vi "Recording_Main.vi"(8 "error in":errorcluster, 11 "QRD":T1) -> (0 "error out":errorcluster)   [LabVIEW 2025]
uses:
  Builds/Queue Wrappers.lvlibp
  Controls/Local Data_Recording.ctl
  Builds/Queue Wrappers.lvlibp/Q Packet.ctl
  Controls/Queues-Refs-Data.ctl
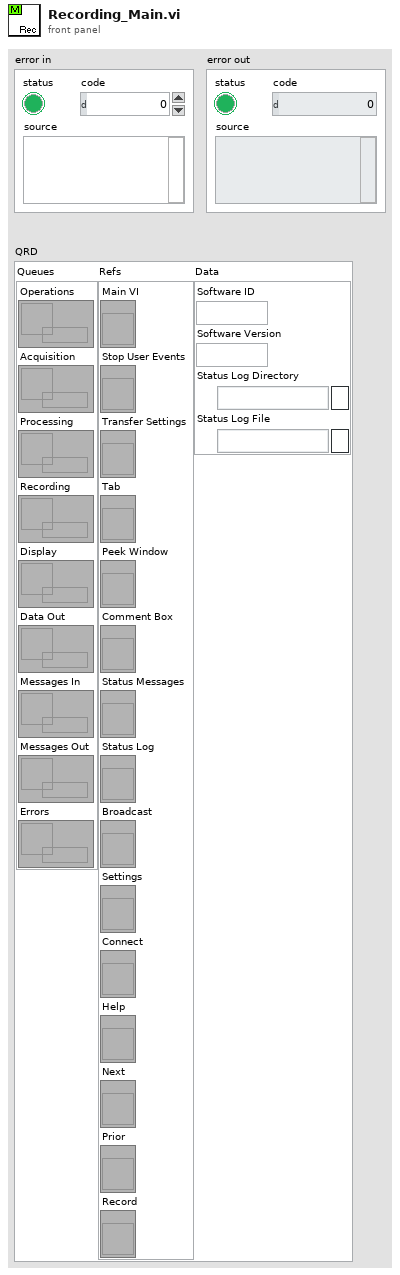
[diagram p1: front panel]
types:
  T1 = typedef "Queues-Refs-Data.ctl" = cluster{"Queues":cluster{"Operations":refnum<queue>, "Acquisition":refnum<queue>, "Processing":refnum<queue>, "Recording":refnum<queue>, "Display":refnum<queue>, "Data Out":refnum<queue>, "Messages In":refnum<queue>, "Messages Out":refnum<queue>, "Errors":refnum<queue>}, "Refs":cluster{"Main VI":refnum<vi>, "Stop User Events":refnum<vi>, "Transfer Settings":refnum<vi>, "Tab":refnum<vi>, "Peek Window":refnum<vi>, "Comment Box":refnum<vi>, "Status Messages":refnum<vi>, "Status Log":refnum<vi>, "Broadcast":refnum<vi>, "Settings":refnum<vi>, "Connect":refnum<vi>, "Help":refnum<vi>, "Next":refnum<vi>, "Prior":refnum<vi>, "Record":refnum<vi>}, "Data":cluster{"Software ID":string, "Software Version":string, "Status Log Directory":path, "Status Log File":path}}
  T2 = typedef "Local Data_Recording.ctl" = cluster{"Loop ID":string, "Output Dir":path, "Output File":path, "Output File Ref":refnum<k34>}
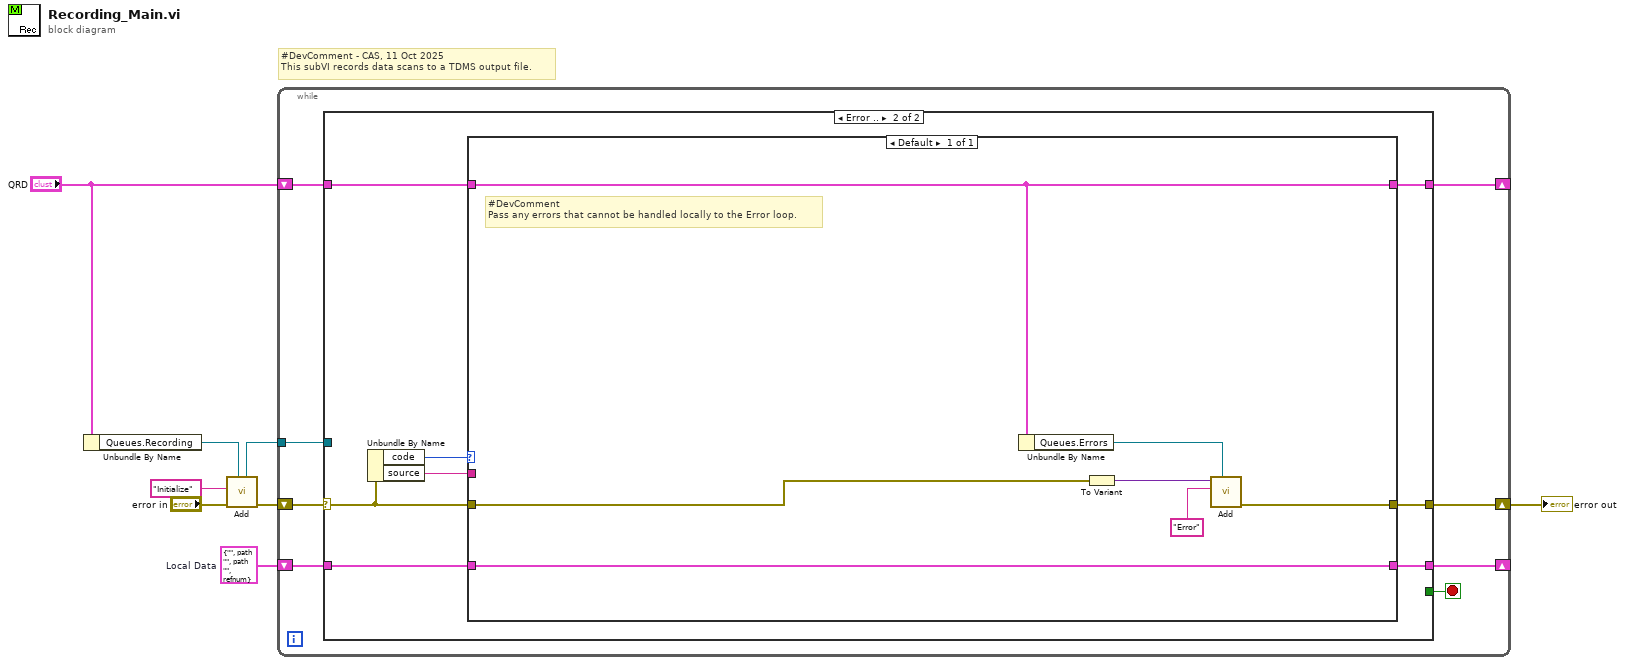
[diagram p0: block diagram]
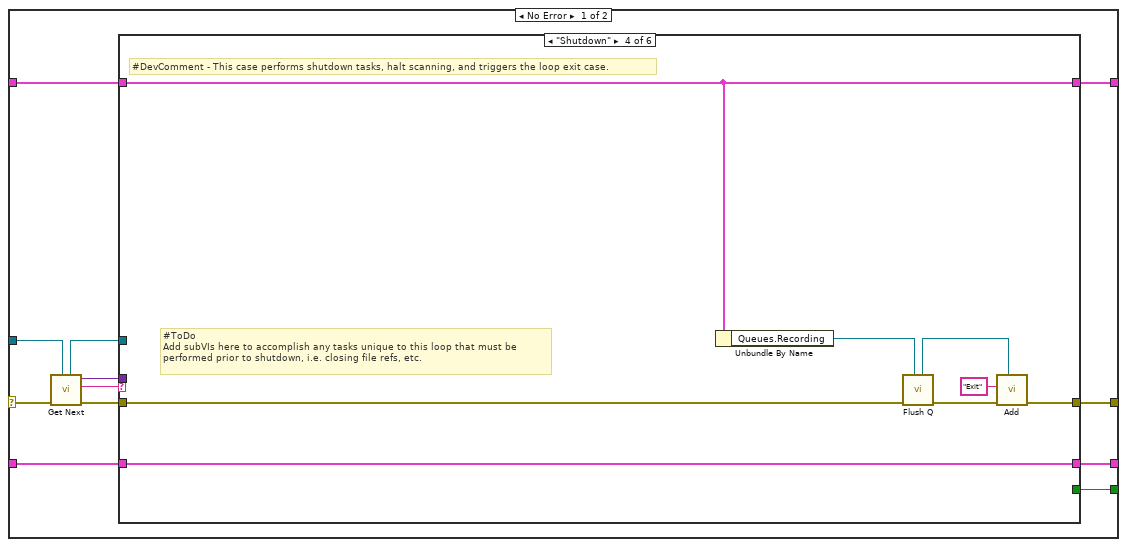
[diagram p2: hidden frame]
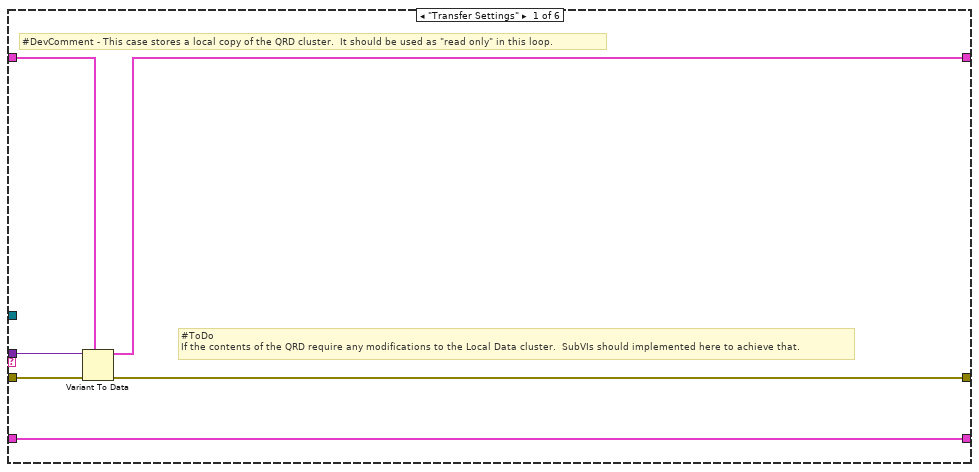
[diagram p3: hidden frame]
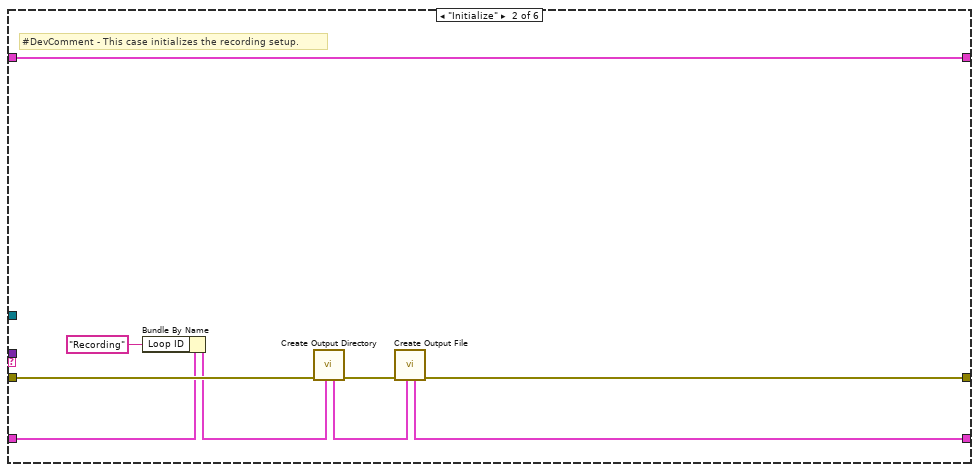
[diagram p4: hidden frame]
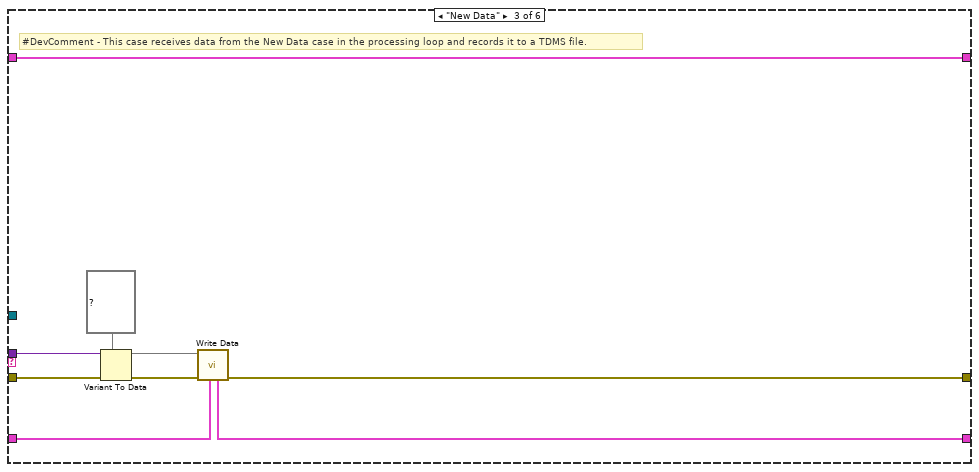
[diagram p5: hidden frame]
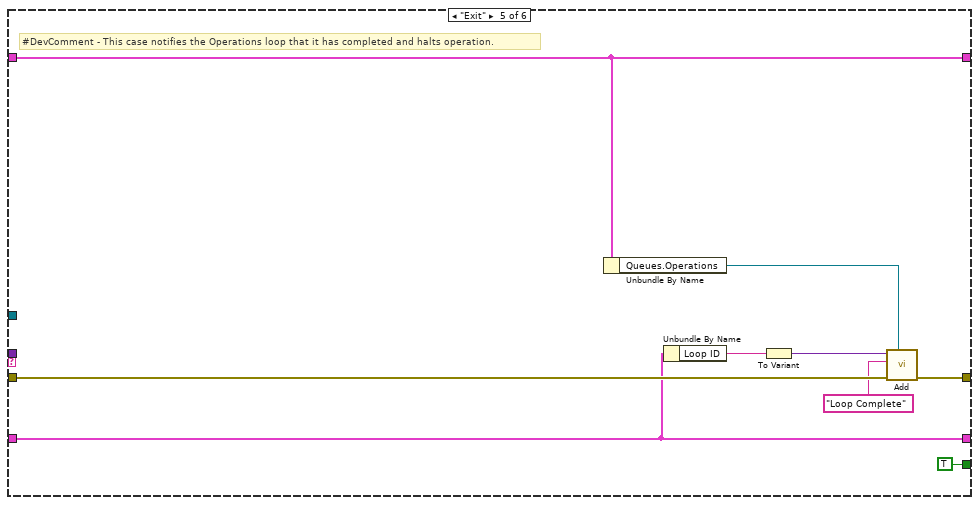
[diagram p6: hidden frame]
diagram:
  w6 = T2 {"Loop ID"="", "Output Dir"=path "", "Output File"=path "", "Output File Ref"=refnum}  # Local Data
  # "#DevComment - CAS, 11 Oct 2025\nThis subVI records data scans to a TDMS output file."
  n1 = Unbundle By Name("QRD") -> ("Queues.Recording"=w3:refnum<queue>)
  n2 = call "Add.vi"("Q Ref In"=w3, "error in"="error in", "Message ID"="Initialize" ("Packet ID")) -> ("error out"=w4:errorcluster, "Q Ref Out"=w2:refnum<queue>)  [unwired: 5 in, 2 out]
  n3 = while {
    shift-right: [w15] -> _
    shift-left: "QRD" -> [w16]
    shift-right: [w13] -> w8
    shift-left: w4 -> [w14]
    tunnel: w2 -> [w12]
    shift-right: [w9] -> _
    shift-left: w6 -> [w11]
    stop <- w10 stop-if-true
    n4 = case shown="Error .." w14 {
      selector: w14 -> [w28 w77]
      tunnel: w16 -> [w25 w74]
      tunnel: [w26 w75] -> w15
      tunnel: [w23 w76] -> w13
      tunnel: w12 -> [w27 _]
      tunnel: w11 -> [w19 w78]
      tunnel: [w18 w73] -> w9
      tunnel: [w17 _] -> w10
      frame No Error {
        n5 = call "Get Next.vi"("Q Ref In"=w27, "error in"=w28) -> ("error out"=w24:errorcluster, "Message ID"=w20:string, "Payload"=w21:variant, "Q Ref Out"=w22:refnum<queue>)  [unwired: 6 in]
        n6 = case shown="\"Shutdown\"" w20 {
          tunnel: [w30 w43 w50 w60 w69 w72] -> w26
          tunnel: w25 -> [w32 w43 w50 w60 w69 w72]
          tunnel: w24 -> [w34 w41 w52 w58 w67 w71]
          tunnel: [w31 w35 w46 w59 w68 w71] -> w23
          tunnel: w22 -> [_ _ _ _ _ _]
          tunnel: w21 -> [w33 _ w51 _ _ _]
          tunnel: w19 -> [w29 w40 w44 w54 w65 w70]
          tunnel: [w29 w36 w45 w54 w65 w70] -> w18
          tunnel: [_ _ _ _ TRUE _] -> w17
          frame "Transfer Settings" {
            # "#ToDo\nIf the contents of the QRD require any modifications to the Local Data cluster.  SubVIs should implemented here to achieve that."
            # "#DevComment - This case stores a local copy of the QRD cluster.  It should be used as \"read only\" in this loop."
            n7 = Variant To Data(error in=w34, type=w32, Variant=w33) -> (data=w30:T1, error out=w31:errorcluster)
          }
          frame "Initialize" {
            # "#DevComment - This case initializes the recording setup."
            n8 = Bundle By Name(cluster=w40, "Loop ID"="Recording") -> (w39:T2)
            n9 = call "Create Output Directory.vi"("Local Data"=w39, "error in"=w41) -> ("error out"=w38:errorcluster, "Local Data Out"=w37:T2)  [unwired: 8 in]
            n10 = call "Create Output File.vi"("Local Data"=w37, "error in"=w38) -> ("error out"=w35:errorcluster, "Local Data Out"=w36:T2)  [unwired: 8 in]
          }
          frame "New Data" {
            # "#DevComment - This case receives data from the New Data case in the processing loop and records it to a TDMS file."
            n11 = Variant To Data(error in=w52, type=map{string, dbl} {} ("CVT"), Variant=w51) -> (data=w47:map{string, dbl}, error out=w48:errorcluster)
            n12 = call "Write Data.vi"("Local Data"=w44, "error in"=w48, "Current Value Table"=w47) -> ("error out"=w46:errorcluster, "Local Data Out"=w45:T2)  [unwired: 7 in]
          }
          frame "Shutdown" {
            # "#ToDo\nAdd subVIs here to accomplish any tasks unique to this loop that must be\nperformed prior to shutdown, i.e. closing file refs, etc."
            # "#DevComment - This case performs shutdown tasks, halt scanning, and triggers the loop exit case."
            n13 = Unbundle By Name(w60) -> ("Queues.Recording"=w56:refnum<queue>)
            n14 = call "Flush Q.vi"("Q Ref In"=w56, "error in"=w58) -> ("error out"=w57:errorcluster, "Q Ref Out"=w55:refnum<queue>)  [unwired: 7 in, 1 out]
            n15 = call "Add.vi"("Q Ref In"=w55, "error in"=w57, "Message ID"="Exit" ("Packet ID")) -> ("error out"=w59:errorcluster)  [unwired: 5 in, 3 out]
          }
          frame "Exit" {
            # "#DevComment - This case notifies the Operations loop that it has completed and halts operation."
            n16 = Unbundle By Name(w69) -> ("Queues.Operations"=w66:refnum<queue>)
            n17 = Unbundle By Name(w65) -> ("Loop ID"=w64:string)
            n18 = To Variant(anything=w64) -> (Variant=w61:variant)
            n19 = call "Add.vi"("Q Ref In"=w66, "error in"=w67, "Message ID"="Loop Complete" ("Packet ID"), "Payload"=w61) -> ("error out"=w68:errorcluster)  [unwired: 4 in, 3 out]
          }
          frame Default {
          }
        }
      }
      frame Error {
        n20 = Unbundle By Name(w77) -> ("code"=w80:i32, "source"=w79:string)
        n21 = case shown="Default" w80 {
          tunnel: w79 -> [_]
          tunnel: w78 -> [w87]
          tunnel: [w87] -> w73
          tunnel: w77 -> [w83]
          tunnel: [w85] -> w76
          tunnel: [w84] -> w75
          tunnel: w74 -> [w84]
          frame Default {
            # "#DevComment\nPass any errors that cannot be handled locally to the Error loop."
            n22 = Unbundle By Name(w84) -> ("Queues.Errors"=w86:refnum<queue>)
            n23 = To Variant(anything=w83) -> (Variant=w81:variant)
            n24 = call "Add.vi"("Q Ref In"=w86, "Message ID"="Error" ("Packet ID"), "Payload"=w81) -> ("error out"=w85:errorcluster)  [unwired: 5 in, 3 out]
          }
        }
      }
    }
  }
  "error out" <- w8
